vi "FromClusterToTagBusScript.vi"(5 "process":T3={"param?"=TRUE, "Parameter Data Interface VI (blank=tag bus to parameters.vi)"="", "Result Data Interface VI (blank=results to tag bus.vi)"="", "reverse param?"=FALSE, "Rev. Result Interface VI (blank=results from tag bus.vi)"="", "Rev. Parameter Interface VI (blank=tag bus from parameters.vi)"="", "result?"=TRUE, "reverse result?"=FALSE}, 6 "application reference (local)":refnum<vi>, 7 "output":T2={"enable?"=TRUE, "Data Interface VI (blank=tag bus to outputs.vi)"="", "Reverse Interface VI (blank=tag bus from outputs.vi)"="", "reverse?"=FALSE}, 8 "error in":errorcluster, 9 "configuration class path":path, 10 "input":T1={"enable?"=TRUE, "Data Interface VI (blank=input to tag bus.vi)"="", "reverse?"=FALSE, "Reverse Interface VI (blank=input from tag bus.vi)"=""}, 11 "runtime class path":path) -> (0 "error out":errorcluster)   [LabVIEW 2013, in "control module data interface generator.lvlib"]
doc: "THis Vi scripts the index cluster and the VI to convert from a cluster into Tagbus"
uses:
  control module data interface generator.lvlib
  Controls/input script control.ctl
  Controls/output script control.ctl
  Controls/processing script control.ctl
  Controls/ControlsProperties.ctl
  <vilib>/Utility/miscctls.llb/LVPointTypeDef.ctl
  Controls/StateCluster.ctl
  Controls/initialized references.ctl
  Controls/interface VI type.ctl
panel:
  # "Use this tool to update a User Control Module any time a change occurs to any of it's Input, Processing, Results, or Output clusters of channel data. A modification includes adding or removing channels, changing a channel name, or changing a data type.\n\nSpecify the path of both the runtime and configuration classes of the User Control Module and run the VI to create an updated version.\n\nMake sure the specified User Control Module is not loaded in memory before running this script."
  # "These settings determine which interfaces to script. If you have changed the names of your interface VIs you will have to specify the new VI names.\n\nEnabling a given boolean indicates you wish to script a function for that operation. \"Reverse\" operations are quite literally the opposite of normal operations. For example if \"output\" would normally require conversion from the tag bus into custom data, \"reverse\" would provide the interface for generating a tag bus from custom data. This can be useful for debugging."
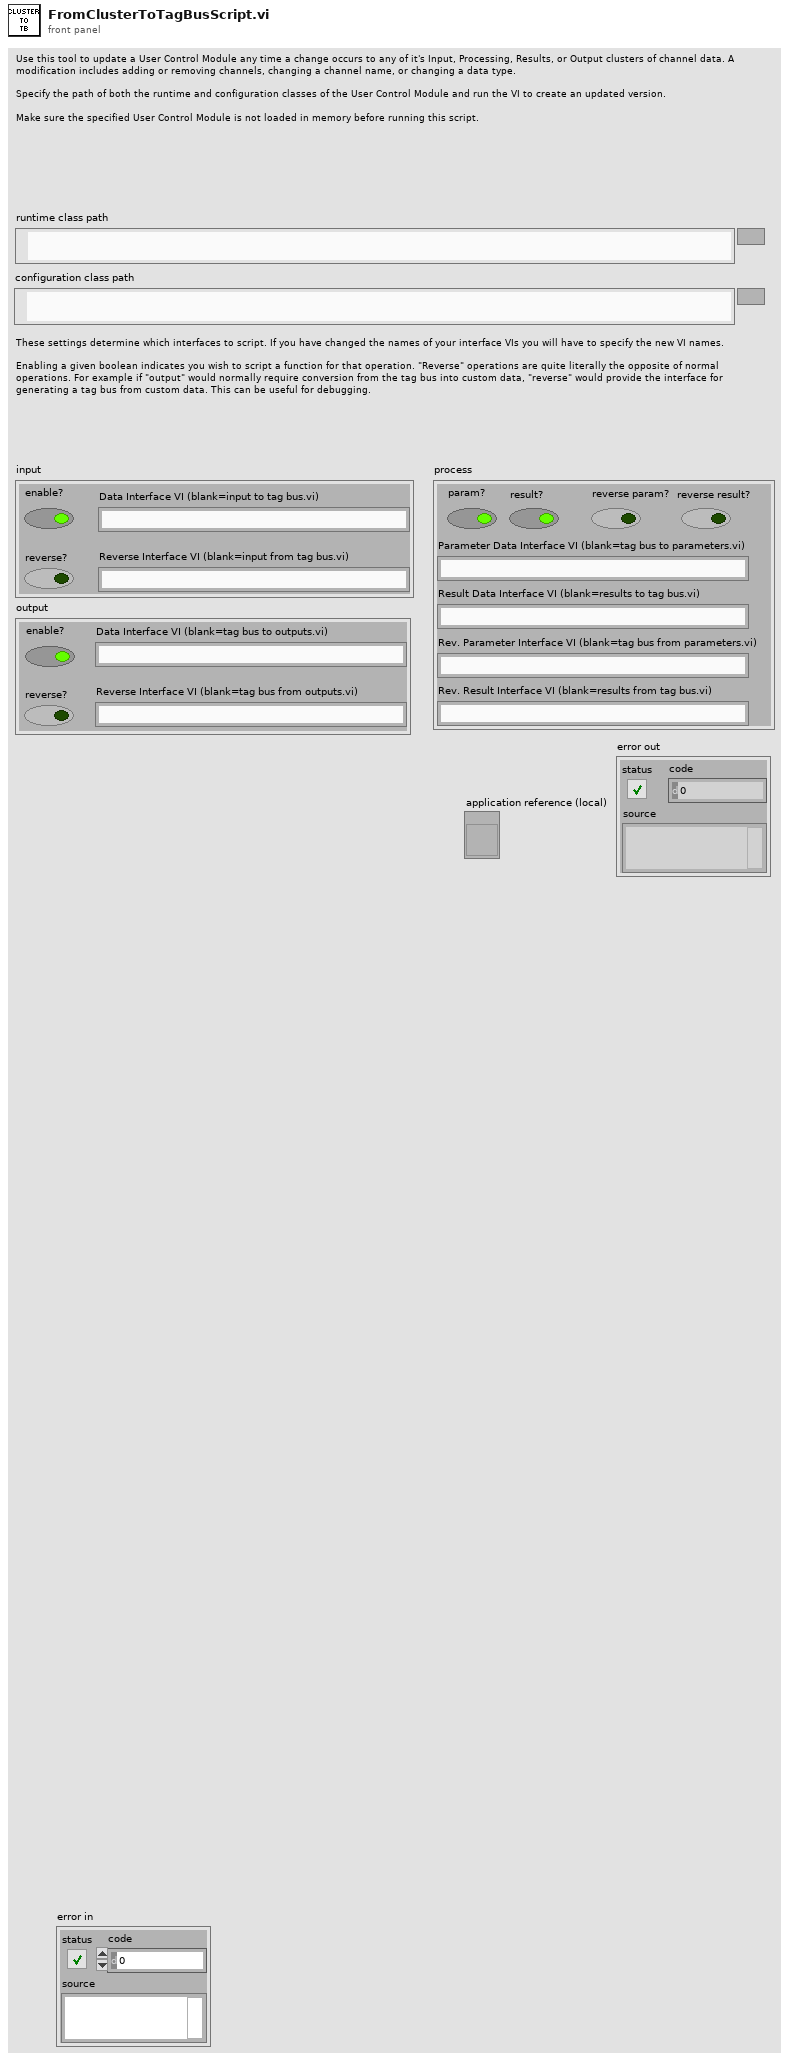
[diagram p1: front panel]
types:
  T1 = typedef "control module data interface generator.lvlib/input script control.ctl" = cluster{"enable?":bool, "Data Interface VI (blank=input to tag bus.vi)":string, "reverse?":bool, "Reverse Interface VI (blank=input from tag bus.vi)":string}
  T2 = typedef "control module data interface generator.lvlib/output script control.ctl" = cluster{"enable?":bool, "Data Interface VI (blank=tag bus to outputs.vi)":string, "Reverse Interface VI (blank=tag bus from outputs.vi)":string, "reverse?":bool}
  T3 = typedef "control module data interface generator.lvlib/processing script control.ctl" = cluster{"param?":bool, "Parameter Data Interface VI (blank=tag bus to parameters.vi)":string, "Result Data Interface VI (blank=results to tag bus.vi)":string, "reverse param?":bool, "Rev. Result Interface VI (blank=results from tag bus.vi)":string, "Rev. Parameter Interface VI (blank=tag bus from parameters.vi)":string, "result?":bool, "reverse result?":bool}
  T4 = typedef "control module data interface generator.lvlib/ControlsProperties.ctl" = cluster{"label":string, "terminal index":u32, "indicator":bool, "location":T5}
  T5 = typedef "LVPointTypeDef.ctl" = cluster{"Horizontal":i16, "Vertical":i16}
  T6 = typedef "control module data interface generator.lvlib/scripting spec.ctl" = cluster{"channel classification":T7, "reverse?":bool, "interface vi":string}
  T7 = typedef "TBM channel.lvclass/channel classification.ctl" = enum16{"input data", "output data", "processing parameter", "processing result"}
  T8 = typedef "owning references.ctl" = cluster{"runtime class ref":refnum<vi>, "breaking control runtime":refnum<vi>, "config class ref":refnum<vi>, "breaking control config":refnum<vi>}
  T9 = typedef "control module data interface generator.lvlib/initialized references.ctl" = cluster{"data ctl":refnum<vi>, "index ctl":refnum<vi>, "interface vi":refnum<vi>, "vi type":T10}
  T10 = typedef "control module data interface generator.lvlib/interface VI type.ctl" = enum16{"tb to data", "data to tb"}
  T11 = typedef "control module data interface generator.lvlib/StateCluster.ctl" = cluster{"base cluster":variant, "vi refs":T9}
  T12 = typedef "control module data interface generator.lvlib/TerminalReferences.ctl" = cluster{"Cluster":refnum<vi>, "Index Cluster":refnum<vi>, "tag bus in":refnum<vi>, "tag bus out":refnum<vi>}
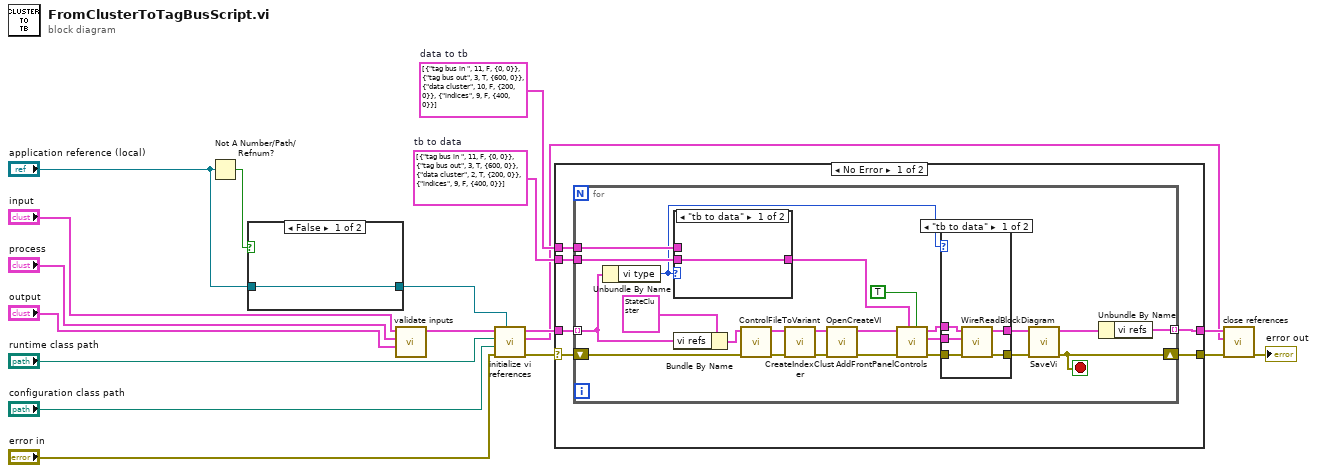
[diagram p0: block diagram]
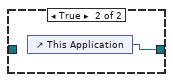
[diagram p2: hidden frame]
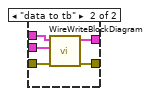
[diagram p3: hidden frame]
diagram:
  w7 = T4[] [{"label"="tag bus in ", "terminal index"=11, "indicator"=FALSE, "location"={"Horizontal"=0, "Vertical"=0}}, {"label"="tag bus out", "terminal index"=3, "indicator"=TRUE, "location"={"Horizontal"=600, "Vertical"=0}}, {"label"="data cluster", "terminal index"=10, "indicator"=FALSE, "location"={"Horizontal"=200, "Vertical"=0}}, {"label"="indices", "terminal index"=9, "indicator"=FALSE, "location"={"Horizontal"=400, "Vertical"=0}}]  # data to tb
  w8 = T4[] [{"label"="tag bus in ", "terminal index"=11, "indicator"=FALSE, "location"={"Horizontal"=0, "Vertical"=0}}, {"label"="tag bus out", "terminal index"=3, "indicator"=TRUE, "location"={"Horizontal"=600, "Vertical"=0}}, {"label"="data cluster", "terminal index"=2, "indicator"=TRUE, "location"={"Horizontal"=200, "Vertical"=0}}, {"label"="indices", "terminal index"=9, "indicator"=FALSE, "location"={"Horizontal"=400, "Vertical"=0}}]  # tb to data
  n1 = Not A Number/Path/Refnum?(number/path/refnum="application reference (local)") -> (NaN/Path/Refnum?=w3:bool)
  n2 = case shown="False" w3 {
    tunnel: [w19 w20] -> w2
    tunnel: "application reference (local)" -> [w19 _]
    frame False {
    }
    frame True {
      n3 = control-ref of="This Application"() -> (w20:refnum<vi>)
    }
  }
  n4 = call "validate inputs.vi"("output in"="output", "process in"="process", "input in"="input") -> ("spec"=w15:T6[])  [unwired: 8 in]
  n5 = call "initialize vi references.vi"("application reference (local)"=w2, "error in"="error in", "config class path"="configuration class path", "runtime class path"="runtime class path", "spec"=w15) -> ("error out"=w14:errorcluster, "owning references"=w4:T8, "initialized references"=w13:T9[])  [unwired: 4 in]
  n6 = case shown="No Error" w14 {
    selector: w14 -> [w25 w63]
    tunnel: w13 -> [w26 w62]
    tunnel: [w24 w63] -> w10
    tunnel: [w21 w62] -> w11
    tunnel: w8 -> [w23 _]
    tunnel: w7 -> [w22 _]
    frame No Error {
      n7 = for {
        tunnel: w26 -> [w46] mode=indexing
        shift-right: [w27] -> w24
        shift-left: w25 -> [w44]
        tunnel: w23 -> [w49]
        tunnel: w22 -> [w48]
        tunnel: [w28] -> w21 mode=indexing
        stop <- w27 stop-if-true
        n8 = Unbundle By Name(w46) -> ("vi type"=w35:T10)
        n9 = case shown="\"tb to data\"" w35 {
          tunnel: [w60 w61] -> w37
          tunnel: w49 -> [w60 _]
          tunnel: w48 -> [_ w61]
          frame "tb to data" {
          }
          frame "data to tb" {
          }
        }
        n10 = Bundle By Name(cluster=T11 {"base cluster"=variant, "vi refs"={"data ctl"=refnum, "index ctl"=refnum, "interface vi"=refnum, "vi type"=enum."tb to data"}} ("State"), "vi refs"=w46) -> (w45:T11)
        n11 = call "ControlFileToVariant.vi"("error in"=w44, "State"=w45) -> ("error out"=w42:errorcluster, "State out"=w43:T11)  [unwired: 8 in]
        n12 = call "CreateIndexCluster.vi"("error in"=w42, "State"=w43) -> ("error out"=w40:errorcluster, "State out"=w41:T11)  [unwired: 8 in]
        n13 = call "OpenCreateVI.vi"("error in"=w40, "State"=w41) -> ("error out"=w39:errorcluster, "State out"=w38:T11)  [unwired: 8 in]
        n14 = call "AddFrontPanelControls.vi"("Open Front Panel"=TRUE, "Control Properties"=w37, "error in"=w39, "State"=w38) -> ("error out"=w32:errorcluster, "Terminal References"=w33:T12, "State out"=w34:T11)  [unwired: 5 in]
        n15 = case shown="\"tb to data\"" w35 {
          tunnel: w34 -> [w54 w59]
          tunnel: w33 -> [w53 w58]
          tunnel: w32 -> [w52 w57]
          tunnel: [w51 w56] -> w30
          tunnel: [w50 w55] -> w31
          frame "tb to data" {
            n16 = call "WireReadBlockDiagram.vi"("error in"=w52, "Terminal References"=w53, "State"=w54) -> ("error out"=w51:errorcluster, "State out"=w50:T11)  [unwired: 7 in]
          }
          frame "data to tb" {
            n17 = call "WireWriteBlockDiagram.vi"("error in"=w57, "Terminal References"=w58, "State"=w59) -> ("error out"=w56:errorcluster, "State out"=w55:T11)  [unwired: 7 in]
          }
        }
        n18 = call "SaveVi.vi"("error in"=w30, "State"=w31) -> ("error out"=w27:errorcluster, "State out"=w29:T11)  [unwired: 8 in]
        n19 = Unbundle By Name(w29) -> ("vi refs"=w28:T9)
      }
    }
    frame Error {
    }
  }
  n20 = call "close references.vi"("error in"=w10, "owning references"=w4, "initialized references"=w11) -> ("error out"=→"error out":errorcluster)  [unwired: 8 in]
